vi "Request Data JSON.vi"(8 "error in (no error)":errorcluster, 11 "GetSceneItemID in":refnum<class "GetSceneItemID.lvclass">) -> (0 "error out":errorcluster, 2 "Request Data JSON":string, 3 "GetSceneItemID out":refnum<class "GetSceneItemID.lvclass">)   [LabVIEW 2022 SP3, in "obs-websocket-lv.lvlib" / "GetSceneItemID.lvclass"]
uses:
  GetSceneItemID.lvclass
  GetSceneItemID.lvclass/GetSceneItemID.ctl
  <vilib>/IlluminatedG/lv-web-crypto/lv-json/JSON/JSON.lvlib
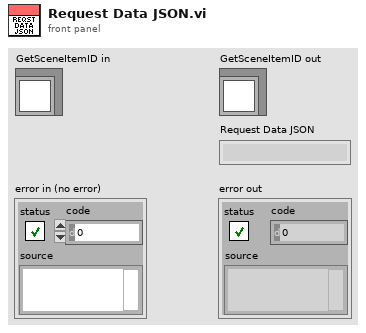
[diagram p1: front panel]
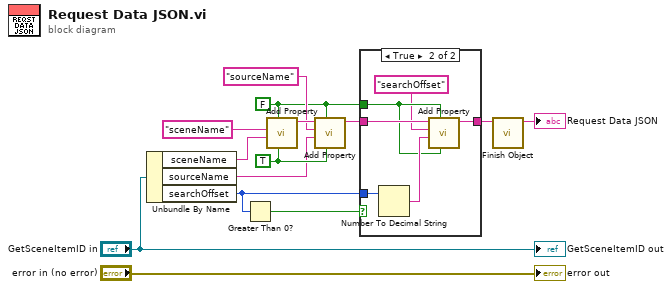
[diagram p0: block diagram]
diagram:
  w3 = FALSE ("Include Empty?")
  w10 = TRUE ("String?")
  n1 = Unbundle By Name("GetSceneItemID in") -> ("sceneName"=w8:string, "sourceName"=w7:string, "searchOffset"=w5:i32)
  n2 = Greater Than 0?(x=w5) -> (x > 0?=w4:bool)
  n3 = call <vilib>:"Add Property.vi"("String?"=w10, "Include Empty?"=w3, "Value"=w8, "Property Name"="sceneName") -> ("String out"=w12:string)  [unwired: 7 in]
  n4 = call <vilib>:"Add Property.vi"("String?"=w10, "Include Empty?"=w3, "Value"=w7, "Property Name"="sourceName", "String In"=w12) -> ("String out"=w6:string)  [unwired: 6 in]
  n5 = case shown="True" w4 {
    tunnel: w6 -> [w15 w21]
    tunnel: w5 -> [_ w20]
    tunnel: w3 -> [_ w18]
    tunnel: [w15 w16] -> w2
    frame False {
    }
    frame True {
      n6 = Number To Decimal String(number=w20) -> (decimal integer string=w19:string)  [unwired: 1 in]
      n7 = call <vilib>:"Add Property.vi"("String?"=w18, "Include Empty?"=w18, "Value"=w19, "Property Name"="searchOffset", "String In"=w21) -> ("String out"=w16:string)  [unwired: 6 in]
    }
  }
  n8 = call <vilib>:"Finish Object.vi"("String In"=w2) -> ("String out"=→"Request Data JSON":string)  [unwired: 10 in]
  "error out" <- "error in (no error)"
  "GetSceneItemID out" <- "GetSceneItemID in"
